vi "cmd_template.vi"(8 "error in (no error)":errorcluster, 11 "JSON":string) -> (0 "error out":errorcluster)   [LabVIEW 2021]
doc: "Command template VI.\n\nWhen you want to create a new command, please copy and modify this VI.\nThe command vi should be placed in the host/cmd directory."
panel:
  in  "args":cluster{"Numeric":dbl}
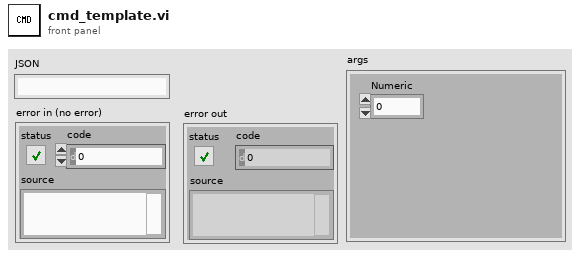
[diagram p1: front panel]
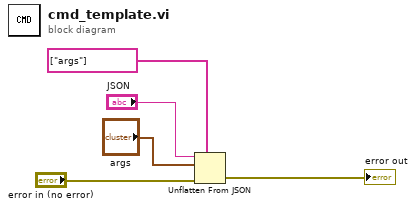
[diagram p0: block diagram]
diagram:
  n1 = Unflatten From JSON(path=string[] ["args"], JSON string="JSON", type and defaults="args", error in (no error)="error in (no error)") -> (error out=→"error out":errorcluster)  [unwired: 3 in, 1 out]
